vi "Get Instrument Alias.vi"(8 "error in (no error)":errorcluster, 11 "DMM6500 in":refnum<class "DMM6500.lvclass">) -> (0 "error out":errorcluster, 2 "Instrument Alias":string, 3 "DMM6500 out":refnum<class "DMM6500.lvclass">)   [LabVIEW 2023, in "HAF.lvlib" / "DMM6500.lvclass"]
doc: "Returns the alias name of the Instrument for this Driver that can be used to initiate a session. Must be implemented by Subclasses because there is no Visa Session available to obtain it from when it is needed.\n\nIt's not ideal: need to think of a better way of dealing with attached resources than hard-coded aliases which must match what was entered in NI-MAX."
uses:
  DMM6500.lvclass
  DMM6500.lvclass/DMM6500.ctl
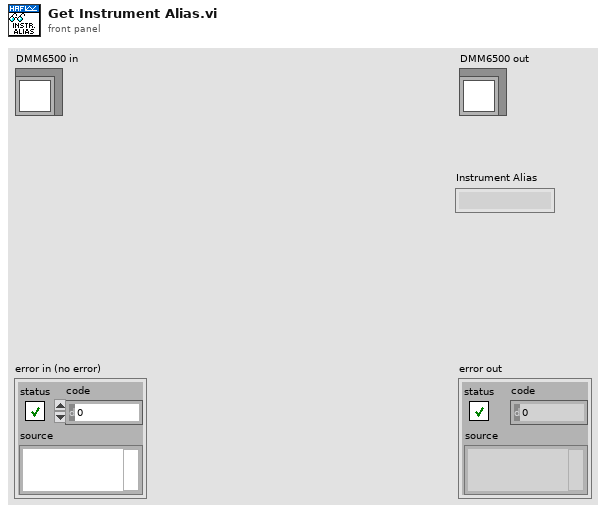
[diagram p1: front panel]
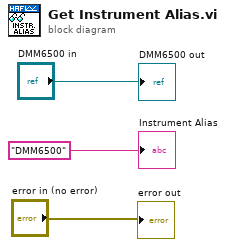
[diagram p0: block diagram]
diagram:
  "error out" <- "error in (no error)"
  "DMM6500 out" <- "DMM6500 in"
  "Instrument Alias" <- "DMM6500" ("Instrument Alias")
